vi "thingspeak.vi"(9 "Data to Post":dbl, 11 "API Key":string="api_key=") -> ()   [LabVIEW 2014]
uses:
  <vilib>/httpClient/POSTBuffer.vi
  <vilib>/httpClient/LabVIEWHTTPClient.lvlib
panel:
  out "Post Data":string
  out "Response Header":string
  out "Response Body":string
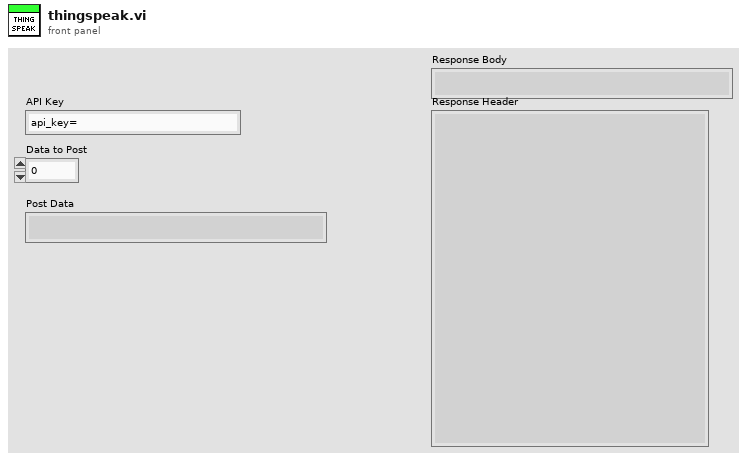
[diagram p1: front panel]
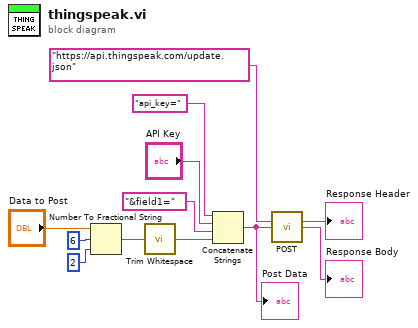
[diagram p0: block diagram]
diagram:
  n1 = Number To Fractional String(number="Data to Post", width (-)=6, precision (6)=2) -> (F-format string=w3:string)  [unwired: 1 in]
  n2 = call <vilib>:"Trim Whitespace.vi"("string"=w3) -> ("trimmed string"=w2:string)  [unwired: 1 in]
  n3 = Concatenate Strings("api_key=", "API Key", "&field1=", w2) -> (w1:string)
  "Post Data" <- w1
  n4 = call-poly <vilib>:"POST.vi"("url"="https://api.thingspeak.com/update.json", "buffer"=w1) -> ("headers"=→"Response Header":string, "body"=→"Response Body":string)  [unwired: 10 in, 2 out]
